vi "Error to Error Log.vi"(8 "error in (no error)":errorcluster, 9 "Previous State":string, 11 "Clear?":bool) -> (0 "error out":errorcluster, 3 "Log Message":string)   [LabVIEW 2011]
doc: "Sends error details to the error log.\n\n\nVersion 1.1 - 6/1/2010\n\nPhaeron, Inc.\nwww.phaeron.net\n\nMatt Whitlock\n303-669-0310"
uses:
  Log Type.ctl
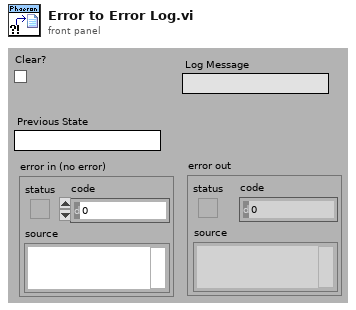
[diagram p1: front panel]
types:
  T1 = typedef "Log Type.ctl" = enum16{"System", "Data", "Error"}
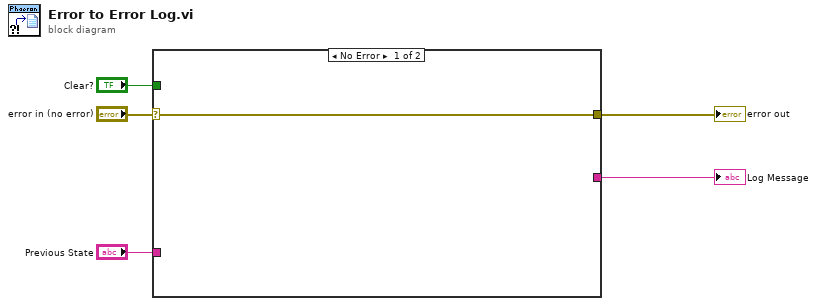
[diagram p0: block diagram]
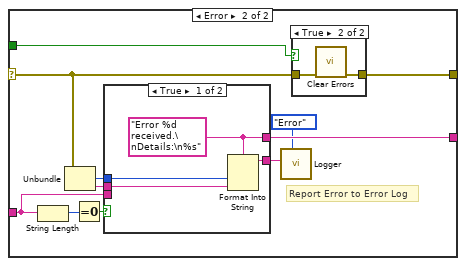
[diagram p2: hidden frame]
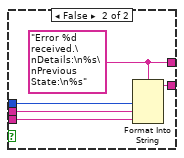
[diagram p3: hidden frame]
diagram:
  n1 = case shown="No Error" "error in (no error)" {
    selector: "error in (no error)" -> [w6 w7]
    tunnel: [w6 w17] -> w5
    tunnel: "Clear?" -> [_ w16]
    tunnel: "Previous State" -> [_ w15]
    tunnel: [_ w9] -> w2
    frame No Error {
    }
    frame Error {
      # "Report Error to Error Log"
      n2 = String Length(string=w15) -> (length=w13:i32)
      n3 = Unbundle(w7) -> ("code"=w12:i32, "source"=w11:string)  [unwired: 1 out]
      n4 = Equal To 0?(x=w13) -> (x = 0?=w14:bool)
      n5 = case shown="True" w14 {
        tunnel: [w21 w26] -> w10
        tunnel: w11 -> [w20 w25]
        tunnel: w12 -> [w19 w24]
        tunnel: [w18 w23] -> w9
        tunnel: w15 -> [_ w22]
        frame True {
          w18 = "Error %d received.\nDetails:\n%s"
          n6 = Format Into String(format string=w18, w19, w20) -> (resulting string=w21:string)  [unwired: 2 in, 1 out]
        }
        frame False {
          w23 = "Error %d received.\nDetails:\n%s\nPrevious State:\n%s"
          n7 = Format Into String(format string=w23, w24, w25, w22) -> (resulting string=w26:string)  [unwired: 2 in, 1 out]
        }
      }
      n8 = call "Logger.vi"("Log Type (System)"=Log_Type."Error", "Information"=w10) -> ()  [unwired: 6 in, 4 out]
      n9 = case shown="True" w16 {
        tunnel: w7 -> [w27 w29]
        tunnel: [w27 w28] -> w17
        frame False {
        }
        frame True {
          n10 = call <vilib>:"Clear Errors.vi"("error in (no error)"=w29) -> ("error out"=w28:errorcluster)  [unwired: 6 in]
        }
      }
    }
  }
  "error out" <- w5
  "Log Message" <- w2
